vi "uA_set_range_uA_mA_shunt_resistor.vi"(8 "error in":errorcluster, 10 "Range - Shunts":T1, 11 "device name":tag="Dev4") -> (0 "error out":errorcluster)   [LabVIEW 2017]
uses:
  Range_Shunt_selector.ctl
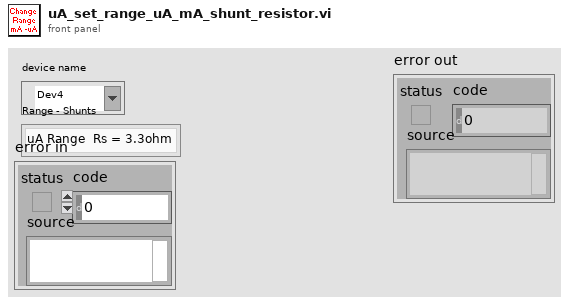
[diagram p1: front panel]
types:
  T1 = typedef "Range_Shunt_selector.ctl" = enum16{"uA Range  Rs = 3.3ohm", "mA Range Rs = 3.3ohm", "mA Range Rs = 1ohm", "mA Range Rs = 1ohm - X2"}
  T2 = enum16{"Set uA Range on Opamp  - Branch 1", "Set mA Range on Opamp - Branch 2"}
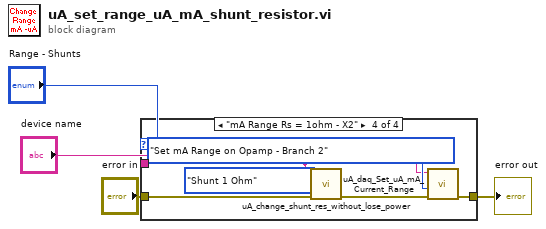
[diagram p0: block diagram]
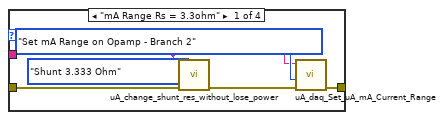
[diagram p2: hidden frame]
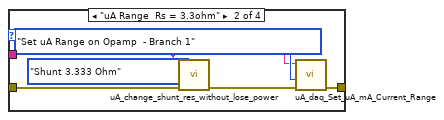
[diagram p3: hidden frame]
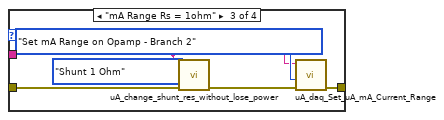
[diagram p4: hidden frame]
diagram:
  n1 = case shown="\"mA Range Rs = 1ohm - X2\"" "Range - Shunts" {
    tunnel: "device name" -> [w7 w11 w19 w25]
    tunnel: "error in" -> [w6 w13 w17 w24]
    tunnel: [w5 w12 w18 w23] -> w1
    frame "mA Range Rs = 3.3ohm" {
      n2 = call "uA_change_shunt_res_without_lose_power.vi"("error in"=w6, "Shunt Slector"=enum16{"Shunt 3.333 Ohm", "Shunt 1 Ohm"}."Shunt 3.333 Ohm", "device name"=w7) -> ("error out"=w8:errorcluster)  [unwired: 8 in]
      n3 = call "uA_daq_Set_uA_mA_Current_Range.vi"("error in"=w8, "Opamp Current Range - Branch 1 & 2"=T2."Set mA Range on Opamp - Branch 2", "device name"=w7) -> ("error out"=w5:errorcluster)  [unwired: 8 in]
    }
    frame "uA Range  Rs = 3.3ohm" {
      n4 = call "uA_change_shunt_res_without_lose_power.vi"("error in"=w13, "Shunt Slector"=enum16{"Shunt 3.333 Ohm", "Shunt 1 Ohm"}."Shunt 3.333 Ohm", "device name"=w11) -> ("error out"=w14:errorcluster)  [unwired: 8 in]
      n5 = call "uA_daq_Set_uA_mA_Current_Range.vi"("error in"=w14, "Opamp Current Range - Branch 1 & 2"=T2."Set uA Range on Opamp  - Branch 1", "device name"=w11) -> ("error out"=w12:errorcluster)  [unwired: 8 in]
    }
    frame "mA Range Rs = 1ohm" {
      n6 = call "uA_change_shunt_res_without_lose_power.vi"("error in"=w17, "Shunt Slector"=enum16{"Shunt 3.333 Ohm", "Shunt 1 Ohm"}."Shunt 1 Ohm", "device name"=w19) -> ("error out"=w20:errorcluster)  [unwired: 8 in]
      n7 = call "uA_daq_Set_uA_mA_Current_Range.vi"("error in"=w20, "Opamp Current Range - Branch 1 & 2"=T2."Set mA Range on Opamp - Branch 2", "device name"=w19) -> ("error out"=w18:errorcluster)  [unwired: 8 in]
    }
    frame "mA Range Rs = 1ohm - X2" {
      n8 = call "uA_change_shunt_res_without_lose_power.vi"("error in"=w24, "Shunt Slector"=enum16{"Shunt 3.333 Ohm", "Shunt 1 Ohm"}."Shunt 1 Ohm", "device name"=w25) -> ("error out"=w26:errorcluster)  [unwired: 8 in]
      n9 = call "uA_daq_Set_uA_mA_Current_Range.vi"("error in"=w26, "Opamp Current Range - Branch 1 & 2"=T2."Set mA Range on Opamp - Branch 2", "device name"=w25) -> ("error out"=w23:errorcluster)  [unwired: 8 in]
    }
  }
  "error out" <- w1
